vi "To Gray_FPGA (SubVI)-RGB.vi"(9 "B":u8, 10 "G":u8, 11 "R":u8) -> (2 "Data Out":u8)   [LabVIEW 2016]
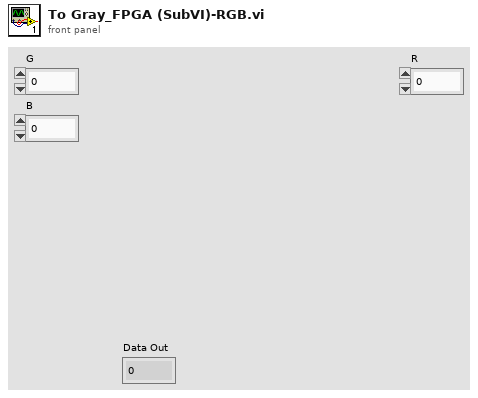
[diagram p1: front panel]
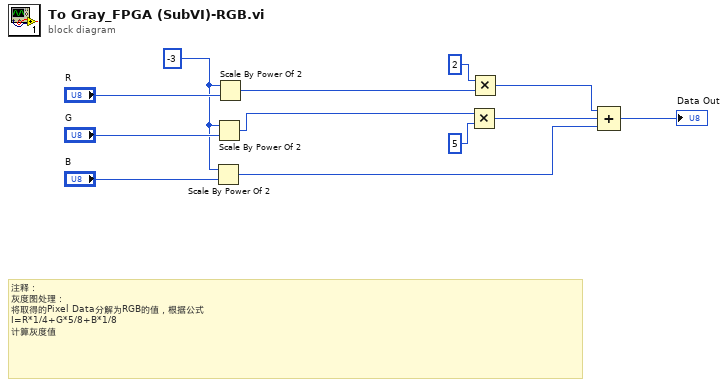
[diagram p0: block diagram]
diagram:
  w9 = i16 -3 ("n")
  # "注释：\n灰度图处理：\n将取得的Pixel Data分解为RGB的值，根据公式\nI=R*1/4+G*5/8+B*1/8\n计算灰度值"
  n1 = Scale By Power Of 2(n=w9, x="B") -> (x*2^n=w7:u8)
  n2 = Scale By Power Of 2(n=w9, x="G") -> (x*2^n=w11:u8)
  n3 = Scale By Power Of 2(n=w9, x="R") -> (x*2^n=w3:u8)
  n4 = Multiply(x=w11, y=u8 5) -> (x*y=w6:u8)
  n5 = Multiply(x=u8 2, y=w3) -> (x*y=w1:u8)
  n6 = Compound Arithmetic op=ADD(w1, w6, w7) -> (→"Data Out":u8)
